vi "Assert Equal Type_Variant.vi"(4 "Execution time (s)":dbl=-1.0, 5 "Assert Only? (F)":bool, 6 "error code (1)":i32=1, 7 "Label":string, 8 "error in (no error)":errorcluster, 10 "Y":variant, 11 "X":variant) -> (0 "error out":errorcluster)   [LabVIEW 2013, in "Caraya.lvlib" / "Assert.lvclass"]
doc: "Generates an error if the input condition is not met.\n\nThis method compares the value of the inputs, irrespective of the type representation.\nAsserts TRUE if input values are equal.\nAsserts FALSE otherwise.\n\nex: Two integer inputs of equal value but of different type representation (U8 and I32) will assert TRUE."
uses:
  Assert.lvclass
panel:
  # "Copyright © 2015 JKI All rights reserved.\n\nAuthor: Tomi Maila <tomi.maila@jki.net>\n\nThis library is provided \"AS IS\" ,WITHOUT WARRANTIES OR\nCONDITIONS OF ANY KIND, either express or implied.\n\nJKI -- jki.net"
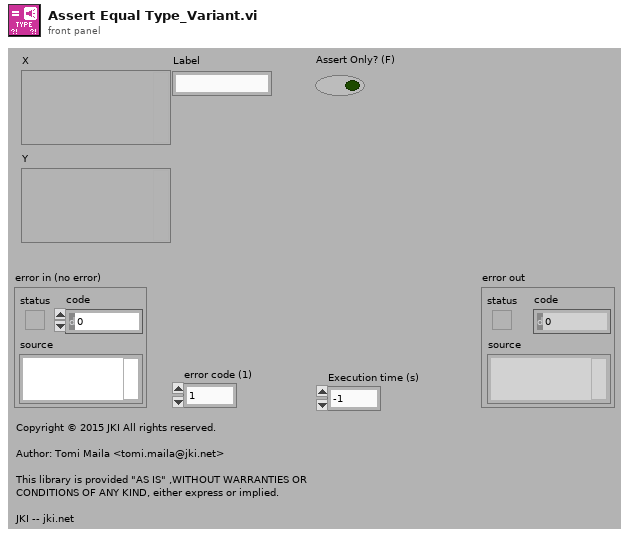
[diagram p1: front panel]
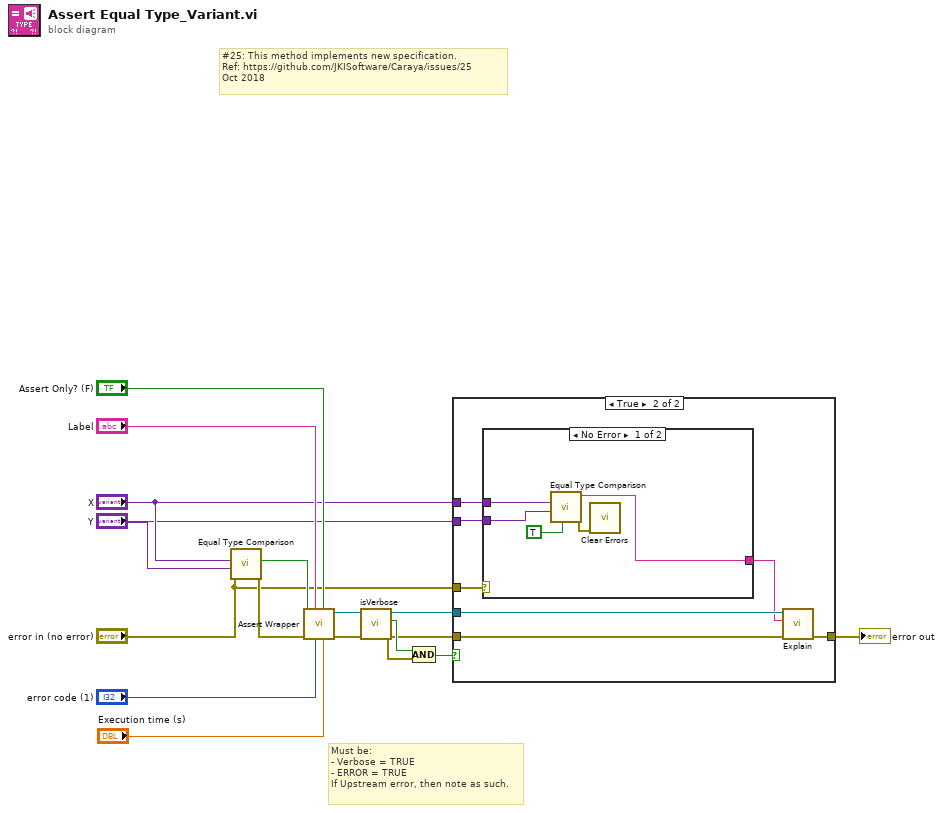
[diagram p0: block diagram]
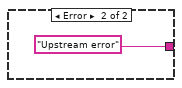
[diagram p3: hidden frame]
diagram:
  # "Must be: \n- Verbose = TRUE\n- ERROR = TRUE\nIf Upstream error, then note as such."
  # "#25: This method implements new specification.\nRef: https://github.com/JKISoftware/Caraya/issues/25\nOct 2018"
  n1 = call "Equal Type Comparison.vi"("error in (no error)"="error in (no error)", "Y"="Y", "X"="X") -> ("error out"=w12:errorcluster, "Equal Types?"=w11:bool)  [unwired: 6 in, 1 out]
  n2 = call "Assert Wrapper.vi"("Execution time (s)"="Execution time (s)", "Assert Only? (F)"="Assert Only? (F)", "error code (1)"="error code (1)", "Label"="Label", "error in (no error)"=w12, "Assert?"=w11) -> ("error out"=w5:errorcluster, "Assert out"=w4:refnum<class "Assert.lvclass">)  [unwired: 4 in]
  n3 = call-dynamic "isVerbose.vi"("Assert in"=w4) -> ("Verbose"=w8:bool, "Assert out"=w9:refnum<class "Assert.lvclass">)  [unwired: 9 in]
  n4 = Compound Arithmetic op=AND(w8, w5) -> (w7:bool)
  n5 = case shown="True" w7 {
    tunnel: [w16 w23] -> w6
    tunnel: w9 -> [_ w22]
    tunnel: w5 -> [w16 w21]
    tunnel: "error in (no error)" -> [_ w20]
    tunnel: "X" -> [_ w18]
    tunnel: "Y" -> [_ w17]
    frame False {
    }
    frame True {
      n6 = case shown="No Error" w20 {
        tunnel: [w25 "Upstream error" ("t")] -> w19
        tunnel: w18 -> [w28 _]
        tunnel: w17 -> [w27 _]
        frame No Error {
          n7 = call "Equal Type Comparison.vi"("verbose? (F)"=TRUE, "Y"=w27, "X"=w28) -> ("error out"=w24:errorcluster, "Verbose output"=w25:string)  [unwired: 6 in, 1 out]
          n8 = call <vilib>:"Clear Errors.vi"("error in (no error)"=w24) -> ()  [unwired: 6 in, 1 out]
        }
        frame Error {
        }
      }
      n9 = call-dynamic "Explain.vi"("error in (no error)"=w21, "Verbose Explanation"=w19, "Assert in"=w22) -> ("error out"=w23:errorcluster)  [unwired: 7 in, 1 out]
    }
  }
  "error out" <- w6
